vi "eGateHSP_LoadDeviceInfo.vi"(7 "path in":path, 8 "Fehler (Eingang, kein Fehler)":errorcluster, 11 "e.gate Configuration":T1 {"StartTime" format="%#.10f"; "dActTimeToSecondFactor" format="%#.10f"; "StartTimeToDayFactor" format="%#_10f"}) -> (0 "Fehler (Ausgang)":errorcluster, 3 "e.gate Configuration 2":T1 {"StartTime" format="%#.10f"; "dActTimeToSecondFactor" format="%#.10f"; "StartTimeToDayFactor" format="%#_10f"})   [LabVIEW 2016]
uses:
  e.gate Configuration.ctl
  e.gate Channel Data.ctl
  e.gate Data Type.ctl
  e.gate Protocol Type.ctl
  e.gate Module  Data.ctl
  e.gateHSP_DLLhandle.ctl
panel:
  out "?":string
  out "?":dbl
  out "?":string
  out "?":dbl
  out "?":string
  out "?":dbl
  out "?":string
  out "?":string
  out "?":dbl
  out "?":string
  out "?":dbl
  out "?":string
  out "?":dbl
  out "?":string
  out "?":dbl
  out "?":dbl
  out "?":dbl
  out "?":string
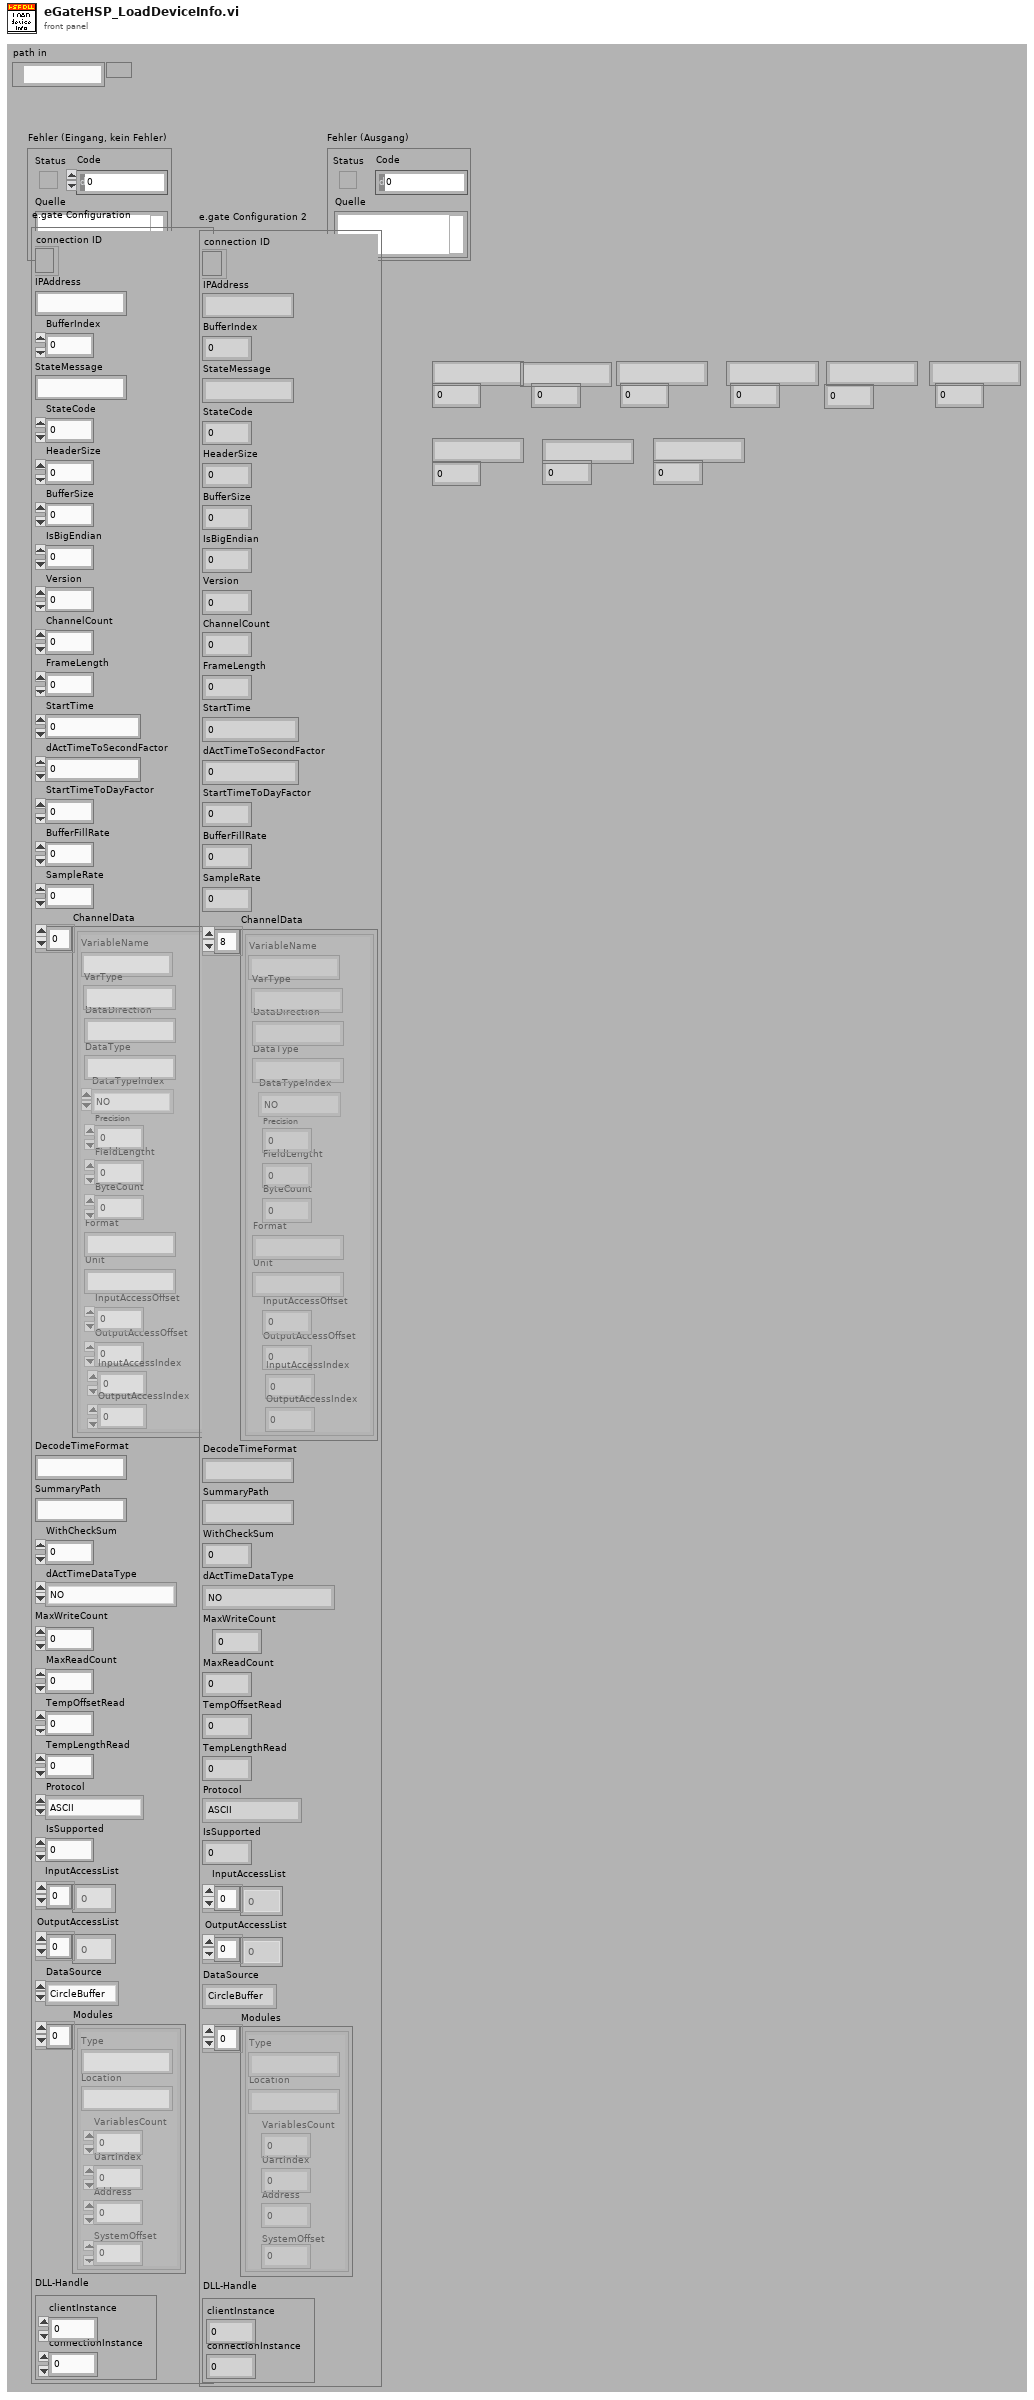
[diagram p1: front panel]
types:
  T1 = typedef "e.gate Configuration.ctl" = cluster{"connection ID":refnum<k5>, "IPAddress":string, "BufferIndex":i32, "StateMessage":string, "StateCode":i8, "HeaderSize":i32, "BufferSize":i32, "IsBigEndian":i32, "Version":i32, "ChannelCount":i32, "FrameLength":i32, "StartTime":dbl, "dActTimeToSecondFactor":dbl, "StartTimeToDayFactor":dbl, "BufferFillRate":dbl, "SampleRate":dbl, "ChannelData":T2[], "DecodeTimeFormat":string, "SummaryPath":string, "WithCheckSum":i32, "dActTimeDataType":T3, "MaxWriteCount":i32, "MaxReadCount":i32, "TempOffsetRead":i32, "TempLengthRead":i32, "Protocol":T4, "IsSupported":i32, "InputAccessList":i32[], "OutputAccessList":i32[], "DataSource":enum16{"CircleBuffer", "test.con Logger", "test.con Archive"}, "Modules":T5[], "DLL-Handle":T6}
  T2 = typedef "e.gate Channel Data.ctl" = cluster{"VariableName":string, "DataDirection":string, "DataType":string, "DataTypeIndex":T3, "Precision":i16, "FieldLengtht":i16, "ByteCount":i32, "Format":string, "Unit":string, "InputAccessOffset":i32, "OutputAccessOffset":i16, "InputAccessIndex":i16, "OutputAccessIndex":i16, "VarType":string}
  T3 = typedef "e.gate Data Type.ctl" = enum16{"NO", "BOOL", "SINT8", "USINT8", "SINT16", "USINT16", "SINT32", "USINT32", "FLOAT", "SET8", "SET16", "SET32", "DOUBLE", "SINT64", "USINT64", "SET64"}
  T4 = typedef "e.gate Protocol Type.ctl" = enum16{"ASCII", "HighspeedPort Online", "HighspeedPort Buffer", "eGateHighspeedPortDLL "}
  T5 = typedef "e.gate Module  Data.ctl" = cluster{"Type":string, "Location":string, "VariablesCount":i16, "UartIndex":i16, "Address":i16, "SystemOffset":i16}
  T6 = typedef "e.gateHSP_DLLhandle.ctl" = cluster{"clientInstance":i32, "connectionInstance":i32}
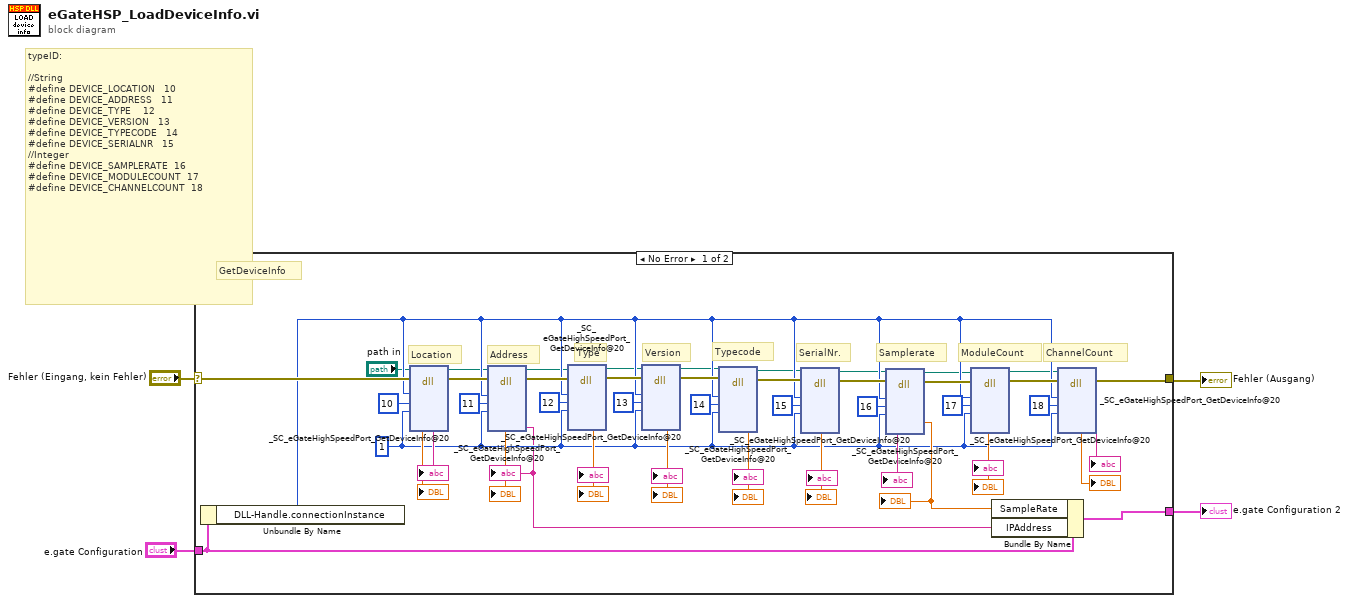
[diagram p0: block diagram]
diagram:
  # "typeID: \n\n//String\n#define DEVICE_LOCATION\t\t\t10\n#define DEVICE_ADDRESS\t\t\t11\n#define DEVICE_TYPE\t\t\t\t12\n#define DEVICE_VERSION\t\t\t13\n#define DEVICE_TYPECODE\t\t\t14\n#define DEVICE_SERIALNR\t\t\t15\n//Integer\n#define DEVICE_SAMPLERATE\t\t16\n#define DEVICE_MODULECOUNT\t\t17\n#define DEVICE_CHANNELCOUNT\t\t18"
  n1 = case shown="No Error" "Fehler (Eingang, kein Fehler)" {
    selector: "Fehler (Eingang, kein Fehler)" -> [w54 w55]
    tunnel: [w39 w55] -> w3
    tunnel: "e.gate Configuration" -> [w15 _]
    tunnel: [w34 _] -> w1
    frame No Error {
      w17 = 1 ("Index")
      # "ChannelCount"
      # "ModuleCount"
      # "Samplerate"
      # "SerialNr."
      # "Typecode"
      # "Version"
      # "Type"
      # "Address"
      # "Location"
      # "GetDeviceInfo"
      n2 = Unbundle By Name(w15) -> ("DLL-Handle.connectionInstance"=w14:i32)
      n3 = dll-call lib="eGateHighSpeedPort.dll" fn="_SC_eGateHighSpeedPort_GetDeviceInfo@20"(path in="path in", error in=w54, "connectionInstance"=w14, "typeID"=10, "Index"=w17) -> (path out=w12:path, error out=w53:errorcluster, "info"=→"?":dbl, "channelInfo"=→"?":string)  [unwired: 7 in]
      n4 = dll-call lib="eGateHighSpeedPort.dll" fn="_SC_eGateHighSpeedPort_GetDeviceInfo@20"(path in=w12, error in=w53, "connectionInstance"=w14, "typeID"=11, "Index"=w17) -> (path out=w11:path, error out=w52:errorcluster, "info"=→"?":dbl, "channelInfo"=w16:string)  [unwired: 7 in]
      "?" <- w16
      n5 = dll-call lib="eGateHighSpeedPort.dll" fn="_SC_eGateHighSpeedPort_GetDeviceInfo@20"(path in=w11, error in=w52, "connectionInstance"=w14, "typeID"=12, "Index"=w17) -> (path out=w10:path, error out=w51:errorcluster, "info"=→"?":dbl, "channelInfo"=→"?":string)  [unwired: 7 in]
      n6 = dll-call lib="eGateHighSpeedPort.dll" fn="_SC_eGateHighSpeedPort_GetDeviceInfo@20"(path in=w10, error in=w51, "connectionInstance"=w14, "typeID"=13, "Index"=w17) -> (path out=w9:path, error out=w50:errorcluster, "info"=→"?":dbl, "channelInfo"=→"?":string)  [unwired: 7 in]
      n7 = dll-call lib="eGateHighSpeedPort.dll" fn="_SC_eGateHighSpeedPort_GetDeviceInfo@20"(path in=w9, error in=w50, "connectionInstance"=w14, "typeID"=14, "Index"=w17) -> (path out=w8:path, error out=w49:errorcluster, "info"=→"?":dbl, "channelInfo"=→"?":string)  [unwired: 7 in]
      n8 = dll-call lib="eGateHighSpeedPort.dll" fn="_SC_eGateHighSpeedPort_GetDeviceInfo@20"(path in=w8, error in=w49, "connectionInstance"=w14, "typeID"=15, "Index"=w17) -> (path out=w7:path, error out=w48:errorcluster, "info"=→"?":dbl, "channelInfo"=→"?":string)  [unwired: 7 in]
      n9 = dll-call lib="eGateHighSpeedPort.dll" fn="_SC_eGateHighSpeedPort_GetDeviceInfo@20"(path in=w7, error in=w48, "connectionInstance"=w14, "typeID"=16, "Index"=w17) -> (path out=w6:path, error out=w47:errorcluster, "info"=w35:dbl, "channelInfo"=→"?":string)  [unwired: 7 in]
      "?" <- w35
      n10 = dll-call lib="eGateHighSpeedPort.dll" fn="_SC_eGateHighSpeedPort_GetDeviceInfo@20"(path in=w6, error in=w47, "connectionInstance"=w14, "typeID"=17, "Index"=w17) -> (path out=w5:path, error out=w40:errorcluster, "info"=→"?":dbl, "channelInfo"=→"?":string)  [unwired: 7 in]
      n11 = Bundle By Name(cluster=w15, "SampleRate"=w35, "IPAddress"=w16) -> (w34:T1)
      n12 = dll-call lib="eGateHighSpeedPort.dll" fn="_SC_eGateHighSpeedPort_GetDeviceInfo@20"(path in=w5, error in=w40, "connectionInstance"=w14, "typeID"=18, "Index"=w17) -> (error out=w39:errorcluster, "info"=→"?":dbl, "channelInfo"=→"?":string)  [unwired: 7 in, 1 out]
    }
    frame Error {
    }
  }
  "Fehler (Ausgang)" <- w3
  "e.gate Configuration 2" <- w1
